vi "getTableRowCellCount.vi"(8 "error in (no error)":errorcluster, 11 "TableRow in":refnum<k24>) -> (0 "error out":errorcluster, 2 "Count":i32, 3 "TableRow out":refnum<k24>)   [LabVIEW 2017, in "LabVIEW NPOI.lvlib" / "xwpfReader.lvclass"]
uses:
  xwpfReader.lvclass
  C:/Users/Neo/Desktop/Dev_Tools_BR/LabVIEW_NPOI/lib/NPOI 2.1.1/NPOI.OOXML.dll
  lib/NPOI 2.1.1/NPOI.OOXML.dll
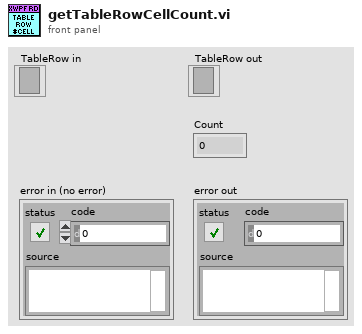
[diagram p1: front panel]
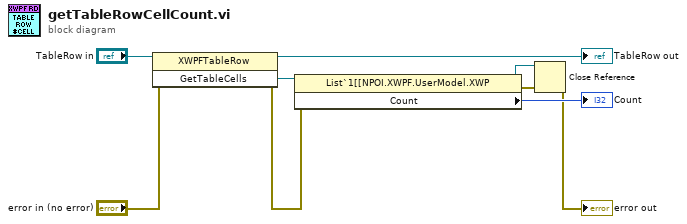
[diagram p0: block diagram]
diagram:
  n1 = invoke class="XWPFTableRow" method="GetTableCells"(reference="TableRow in", error in="error in (no error)") -> (reference out=→"TableRow out":refnum<k24>, error out=w4:errorcluster, "GetTableCells"=w6:refnum<k24>)  [unwired: 1 in]
  n2 = property class="List`1[[NPOI.XWPF.UserModel.XWP"(reference=w6, error in=w4) -> (reference out=w2:refnum<k24>, error out=w3:errorcluster, "Count"=→"Count":i32)
  n3 = Close Reference(reference=w2, error in (no error)=w3) -> (error out=→"error out":errorcluster)
